vi "CMI ADS127L21 - Config Channels.vi"(8 "error in (no error)":errorcluster, 10 "Channels":T1[](array[typedef]) {"Channel" min=1 max=8 step=1}, 11 "session in":T5 {"channels"."Channel" min=1 max=8 step=1}) -> (0 "error out":errorcluster, 3 "session out":T5 {"channels"."Channel" min=1 max=8 step=1})   [LabVIEW 2020]
doc: "Config inputs and select channels for recording from array of channels."
uses:
  CMI ADS127L21 - Session.ctl
  CMI ADS127L21 - Record Channel.ctl
  CMI ADS127L21 - Input Range.ctl
  CMI ADS127L21 - Input Mode.ctl
  CMI ADS127L21 - Input Impedance.ctl
  CMI ADS127L21 - EXTOUT Mode.ctl
  CMI ADS127L21 - EXTOUT Polarity.ctl
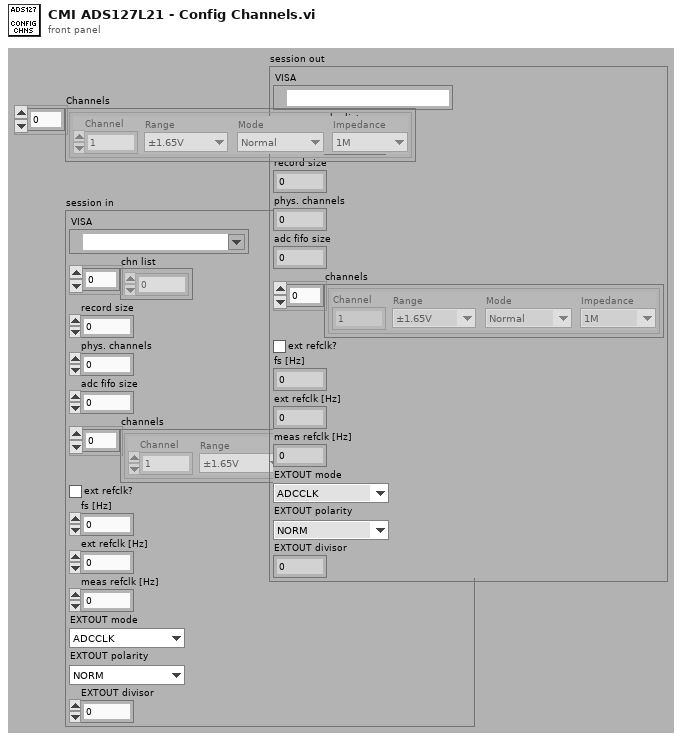
[diagram p1: front panel]
types:
  T1 = typedef "CMI ADS127L21 - Record Channel.ctl" = cluster{"Range":T2, "Channel":i32, "Mode":T3, "Impedance":T4}
  T2 = typedef "CMI ADS127L21 - Input Range.ctl" = enum16{"±1.65V", "±2V"}
  T3 = typedef "CMI ADS127L21 - Input Mode.ctl" = enum16{"Normal", "Inverted", "GND"}
  T4 = typedef "CMI ADS127L21 - Input Impedance.ctl" = enum16{"1M", "1k5"}
  T5 = typedef "CMI ADS127L21 - Session.ctl" = cluster{"VISA":refnum<visa-resource-name>, "chn list":i32[], "record size":i32, "phys. channels":i32, "adc fifo size":i32, "channels":T1[], "ext refclk?":bool, "fs [Hz]":dbl, "ext refclk [Hz]":dbl, "meas refclk [Hz]":dbl, "EXTOUT mode":T6, "EXTOUT polarity":T7, "EXTOUT divisor":i32}
  T6 = typedef "CMI ADS127L21 - EXTOUT Mode.ctl" = enum16{"ADCCLK", "REFCLK", "SMPLCLK", "FIRST"}
  T7 = typedef "CMI ADS127L21 - EXTOUT Polarity.ctl" = enum16{"NORM", "INV"}
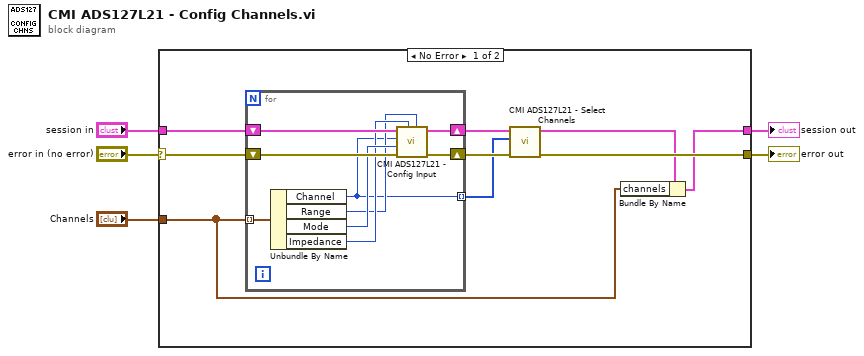
[diagram p0: block diagram]
diagram:
  n1 = case shown="No Error" "error in (no error)" {
    selector: "error in (no error)" -> [w14 w25]
    tunnel: "session in" -> [w13 w24]
    tunnel: [w7 w24] -> w4
    tunnel: [w9 w25] -> w3
    tunnel: "Channels" -> [w6 _]
    frame No Error {
      n2 = for {
        tunnel: w6 -> [w23] mode=indexing
        shift-right: [w16] -> w12
        shift-left: w14 -> [w22]
        shift-right: [w17] -> w11
        shift-left: w13 -> [w21]
        tunnel: [w15] -> w10 mode=indexing
        n3 = Unbundle By Name(w23) -> ("Channel"=w15:i32, "Range"=w18:T2, "Mode"=w20:T3, "Impedance"=w19:T4)
        n4 = call "CMI ADS127L21 - Config Input.vi"("Range"=w18, "Impedance"=w19, "error in (no error)"=w22, "Mode"=w20, "channel id (1: first)"=w15, "session in"=w21) -> ("error out"=w16:errorcluster, "session out"=w17:T5)  [unwired: 4 in]
      }
      n5 = call "CMI ADS127L21 - Select Channels.vi"("error in (no error)"=w12, "Channels List ([1,2])"=w10, "session in"=w11) -> ("error out"=w9:errorcluster, "session out"=w8:T5)  [unwired: 7 in]
      n6 = Bundle By Name(cluster=w8, "channels"=w6) -> (w7:T5)
    }
    frame Error {
    }
  }
  "error out" <- w3
  "session out" <- w4
